vi "Get Status.vi"(8 "error in (no error)":errorcluster, 11 "Executor Reference":refnum<class "Executor.lvclass">) -> (0 "error out":errorcluster, 1 "Safe Shutdown?":bool, 2 "Status[]":T1[](array[typedef]), 3 "Executor Reference":refnum<class "Executor.lvclass">)   [LabVIEW 2014, in "Executor.lvclass"]
uses:
  Executor.lvclass
  Controls/Executor Status - STYP.ctl
  Executor.lvclass/Executor.ctl
  Controls/Executor Data - STYP.ctl
  Controls/Job Results - STYP.ctl
  <vilib>/ActorFramework/Message Enqueuer/Message Enqueuer.lvclass
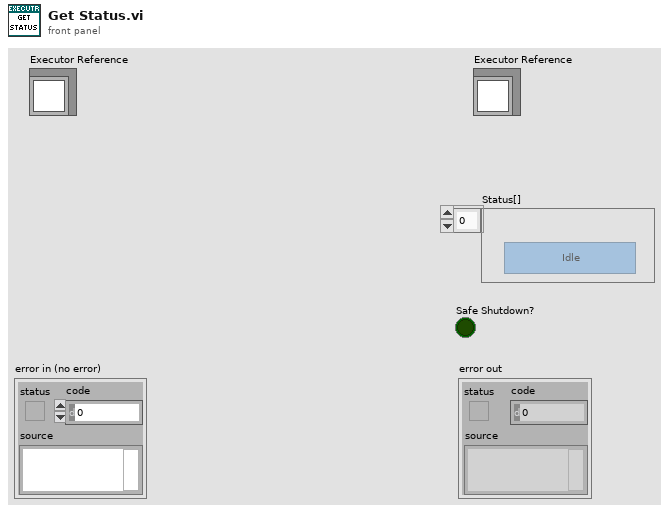
[diagram p1: front panel]
types:
  T1 = typedef "Executor Status - STYP.ctl" = cluster{"Executor Name":string, "Status":bool}
  T2 = typedef "Executor Data - STYP.ctl" = cluster{"Status":T1, "Result Queue":refnum<queue>, "Actor Enquerer":refnum<class "Message Enqueuer.lvclass">}
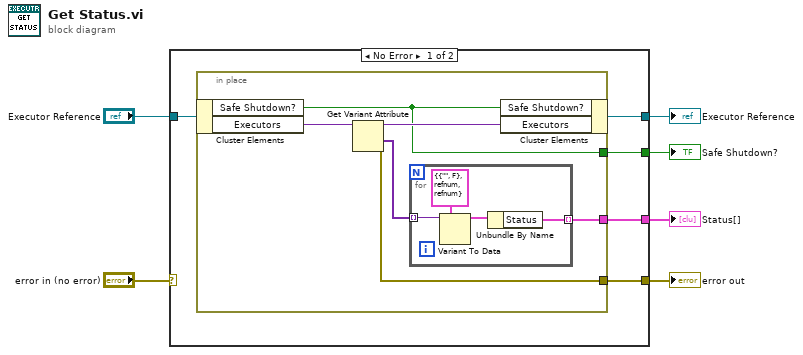
[diagram p0: block diagram]
diagram:
  n1 = case shown="No Error" "error in (no error)" {
    selector: "error in (no error)" -> [_ w23]
    tunnel: [w11 w23] -> w5
    tunnel: [w7 w22] -> w3
    tunnel: "Executor Reference" -> [w8 w22]
    tunnel: [w10 _] -> w2
    tunnel: [w9 _] -> w1
    frame No Error {
      n2 = in-place {
        in-place-border: [w15] -> w11
        in-place-border: [w14] -> w10
        in-place-border: [w13] -> w9
        n3 = in-place-cluster #1(w8) -> ("Safe Shutdown?"=w13:bool, "Executors"=w12:variant)
        n4 = Get Variant Attribute(Variant=w12) -> (duplicate Variant=w17:variant, values=w16:variant[], error out=w15:errorcluster)  [unwired: 3 in, 1 out]
        n5 = for {
          tunnel: w16 -> [w21] mode=indexing
          tunnel: [w18] -> w14 mode=indexing
          n6 = Variant To Data(type=T2 {"Status"={"Executor Name"="", "Status"=FALSE}, "Result Queue"=refnum, "Actor Enquerer"=refnum} ("Executor Data"), Variant=w21) -> (data=w19:T2)  [unwired: 1 in, 1 out]
          n7 = Unbundle By Name(w19) -> ("Status"=w18:T1)
        }
        n8 = in-place-cluster #1("Safe Shutdown?"=w13, "Executors"=w17) -> (w7:refnum<class "Executor.lvclass">)
      }
    }
    frame Error {
    }
  }
  "error out" <- w5
  "Executor Reference" <- w3
  "Status[]" <- w2
  "Safe Shutdown?" <- w1
